vi "sm.main-distance.vi"(10 "y":fxp<+/-,32,2>, 11 "x":fxp<+/-,32,2>) -> (3 "distance":fxp<+/-,32,2>)   [LabVIEW 2019]
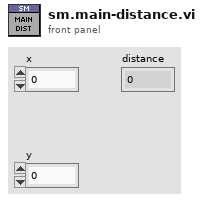
[diagram p1: front panel]
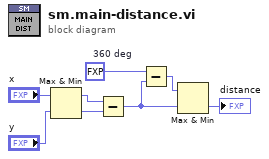
[diagram p0: block diagram]
diagram:
  w1 = fxp<+,1,1> 1.0  # 360 deg
  n1 = Max & Min(x="x", y="y") -> (max(x,y)=w5:fxp<+/-,32,2>, min(x,y)=w4:fxp<+/-,32,2>)
  n2 = Subtract(x=w5, y=w4) -> (x-y=w6:fxp<+/-,32,2>)
  n3 = Subtract(x=w1, y=w6) -> (x-y=w7:fxp<+/-,32,2>)
  n4 = Max & Min(x=w7, y=w6) -> (min(x,y)=→"distance":fxp<+/-,32,2>)  [unwired: 1 out]
